vi "Transmitter_SC - With timer.vi"() -> ()   [LabVIEW 2022 SP3]
uses:
  <instrlib>/niUSRP/niUSRP Write Tx Data (CDB Cluster).vi
panel:
  in  "Iterations":i32=10000
  out "Time(s)":sgl format="%#_4g"
  in  "Alpha":dbl(slide)=0.05 step=0.005 scale=0.0..1.0
  in  "Tab Control":enum32{"USRP Parameters", "Transmission"}(tab)
  in  "USRP ControledParameters 2":T1={"Active Antenna"="TX1", "Gain (dB)"=0.0, "Carrier Frequency"=2400000000.0, "IQ Rate"=2000000.0, "Active Channel"="0"} {"IQ Rate" format="%#_6p"; "Carrier Frequency" format="%#_6p"; "Gain (dB)" format="%#_6f"}
  in  "Device selection":refnum<k15>="RIO0"
  in  "stop":bool
  out "Error out":errorcluster
  in  "Modulation parameter":T2={"Modulation type"=enum."16QAM", "BCC rate (k/n)"=enum."1/2"}
  out "Bits length":i32
  out "Bits length 2":i32
  out "Frame Duration":dbl format="%#_6p"
  out "Coerced Parameters":T3={"IQ Rate"=100000.0, "Carrier  Freq."=100000.0, "Gain"=0.0} {"Gain" format="%#_6f"; "Carrier  Freq." format="%#_6p"; "IQ Rate" format="%#_6p"}
  out "Transmitted Waveform":cluster{"t0":dbl, "dt":dbl, "Y":dbl[]}(graph)
  in  "Message 2":string="ptua. At vero eos et accusam et justo duo dolores et ea rebum. Stet clita kasd gubergren, no sea takimata sanctus est Lorem ipsum dolor sit amet. Lore"
  in  "Message 1":string="Lorem ipsum dolor sit amet, consetetur sadipscing elitr, sed diam nonumy eirmod tempor invidunt ut labore et dolore magna aliquyam erat, sed diam volu"
  in  "error in (no error)":errorcluster
  # "OFDM Superposition Coded Transmitter"
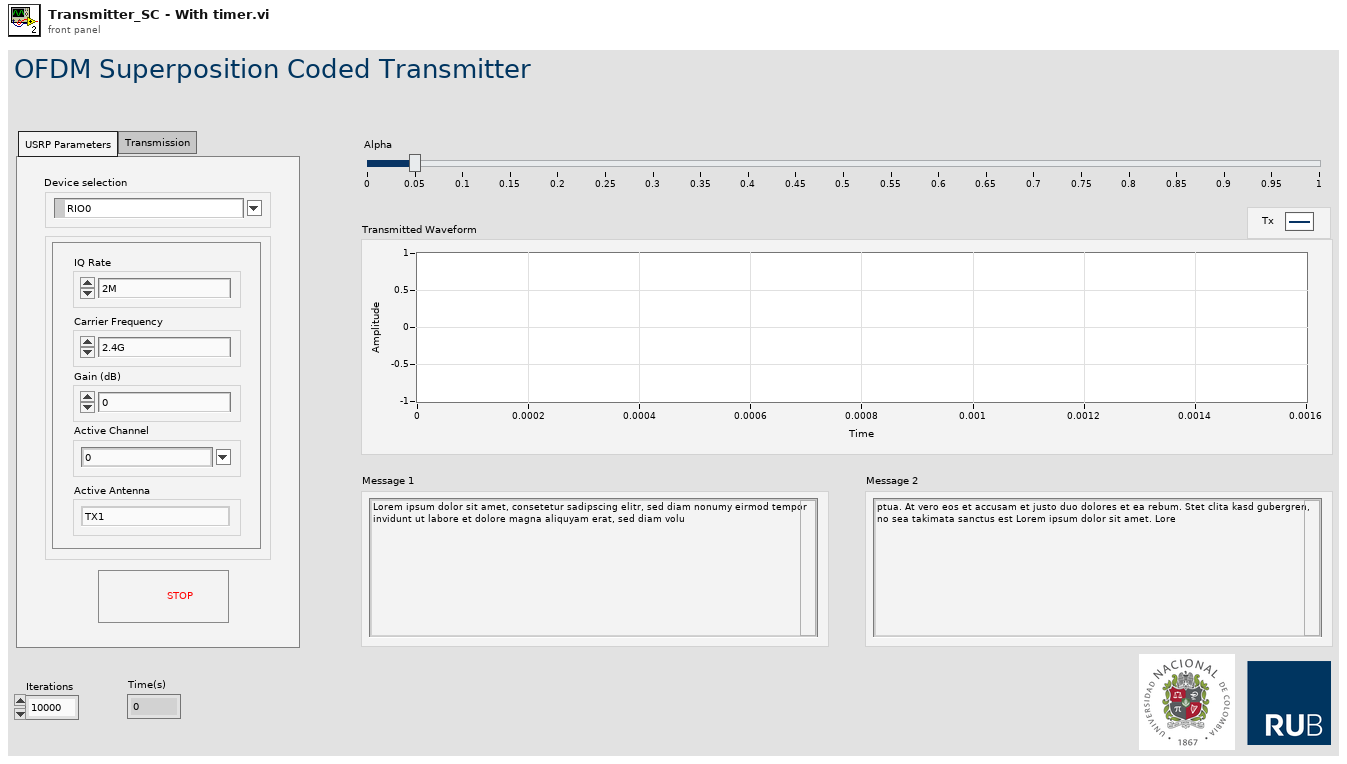
[diagram p1: front panel]
types:
  T1 = cluster{"Active Antenna":string, "Gain (dB)":dbl, "Carrier Frequency":dbl, "IQ Rate":dbl, "Active Channel":string}
  T2 = cluster{"Modulation type":enum16{"QPSK(4QAM)", "64QAM", "16QAM", "BPSK"}, "BCC rate (k/n)":enum16{"1/2", "2/3", "3/4"}}
  T3 = cluster{"IQ Rate":dbl, "Carrier  Freq.":dbl, "Gain":dbl}
  T4 = cluster{"coerced IQ rate":dbl, "coerced carrier frequency":dbl, "coerced gain":dbl}
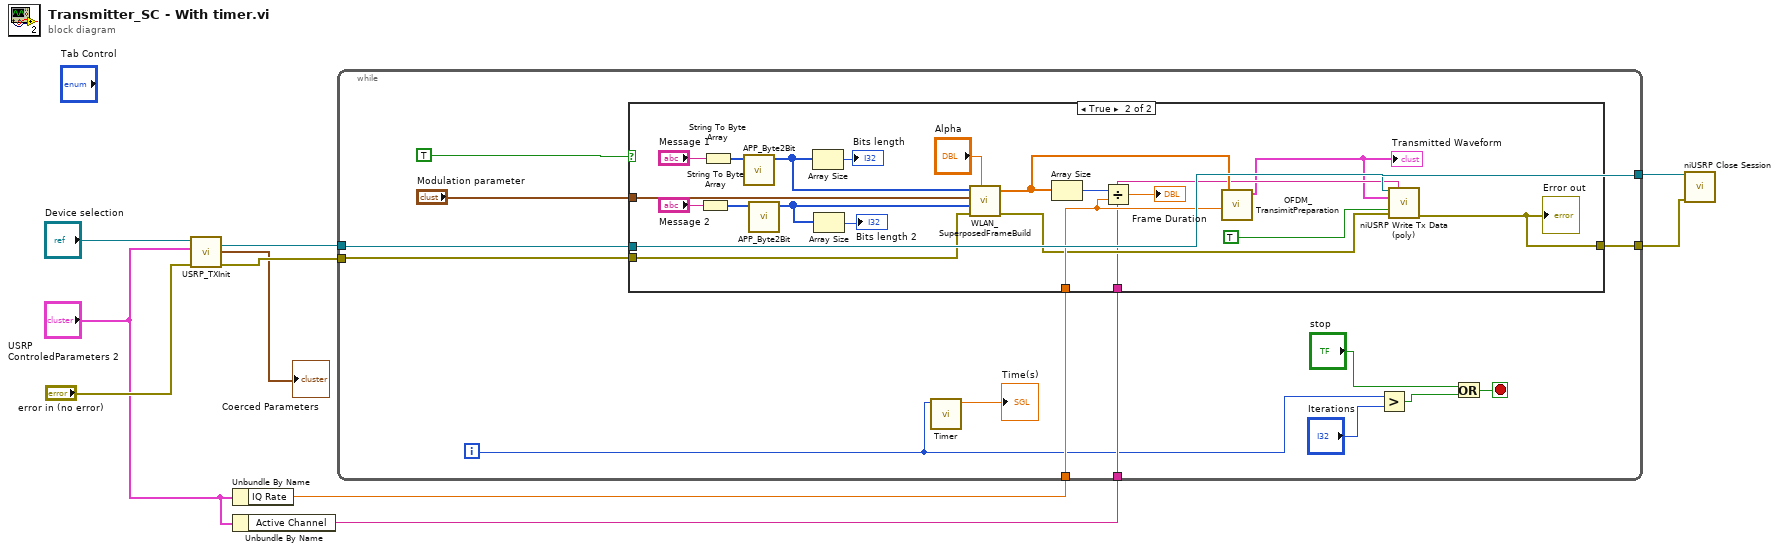
[diagram p0: block diagram]
diagram:
  n1 = call "USRP_TXInit.vi"("device names"="Device selection", "USRP ControledParameters"="USRP ControledParameters 2", "error in (no error)"="error in (no error)") -> ("session handle out"=w9:refnum<k15>, "USRP CoercedParamters"=→"Coerced Parameters":T4, "error out"=w8:errorcluster)  [unwired: 5 in]
  n2 = Unbundle By Name("USRP ControledParameters 2") -> ("IQ Rate"=w7:dbl)
  n3 = Unbundle By Name("USRP ControledParameters 2") -> ("Active Channel"=w1:string)
  n4 = while {
    tunnel: w9 -> [w23]
    tunnel: w8 -> [w21]
    tunnel: w7 -> [w22]
    tunnel: [w23] -> w6
    tunnel: [w20] -> w5
    tunnel: w1 -> [w19]
    i -> [w15]
    stop <- w12 stop-if-true
    n5 = case shown="True" TRUE {
      tunnel: w23 -> [_ w41]
      tunnel: w22 -> [_ w39]
      tunnel: "Modulation parameter" -> [_ w33]
      tunnel: w21 -> [w24 w32]
      tunnel: [w24 w28] -> w20
      tunnel: w19 -> [_ w26]
      frame False {
      }
      frame True {
        n6 = String To Byte Array(string="Message 2") -> (unsigned byte array=w35:u8[])
        n7 = String To Byte Array(string="Message 1") -> (unsigned byte array=w37:u8[])
        n8 = call "APP_Byte2Bit.vi"("input byte stream"=w37) -> ("output bit stream"=w29:i8[])  [unwired: 10 in]
        n9 = call "APP_Byte2Bit.vi"("input byte stream"=w35) -> ("output bit stream"=w34:i8[])  [unwired: 10 in]
        n10 = Array Size(array=w29) -> (size(s)=→"Bits length":i32)
        n11 = Array Size(array=w34) -> (size(s)=→"Bits length 2":i32)
        n12 = call "WLAN_SuperposedFrameBuild.vi"("Alpha"="Alpha", "error in (no error)"=w32, "data in 2"=w34, "Modulation parameter"=w33, "data in"=w29) -> ("error out"=w31:errorcluster, "output array"=w30:cdb[])  [unwired: 5 in]
        n13 = Array Size(array=w30) -> (size(s)=w44:i32)
        n14 = Divide(x=w44, y=w39) -> (x/y=→"Frame Duration":dbl)
        n15 = call "OFDM_TransimitPreparation.vi"("IQ rate"=w39, "array"=w30) -> ("output cluster"=w25:cluster{"t0":dbl, "dt":dbl, "Y":cdb[]})  [unwired: 9 in]
        "Transmitted Waveform" <- w25
        n16 = call-poly <instrlib>:"niUSRP Write Tx Data (poly).vi"("session handle"=w41, "channel list"=w26, "data"=w25, "end of data?"=TRUE, "error in (no error)"=w31) -> ("error out"=w28:errorcluster)  [unwired: 9 in, 1 out]
        "Error out" <- w28
      }
    }
    n17 = call "Timer.vi"("index"=w15) -> ("Time(s)"=→"Time(s)":sgl)  [unwired: 10 in]
    n18 = Greater?(x=w15, y="Iterations") -> (0:w14:bool)
    n19 = Or(x="stop", y=w14) -> (x .or. y?=w12:bool)
  }
  n20 = call <instrlib>:"niUSRP Close Session.vi"("session handle"=w6, "error in (no error)"=w5) -> ()  [unwired: 13 in, 1 out]
